vi "Calc_Waveform.vi"(1 "X-length":dbl, 5 "CamTolerance":dbl=1.1, 9 "frequency in":dbl=5000.0, 11 "error in":errorcluster, 12 "X-Delta":dbl) -> (4 "TriggerLineCamWavepoints":dbl[](array[numeric]), 6 "divisor out":i32, 8 "Array":u8[](array[numeric]), 15 "error out":errorcluster)   [LabVIEW 2011]
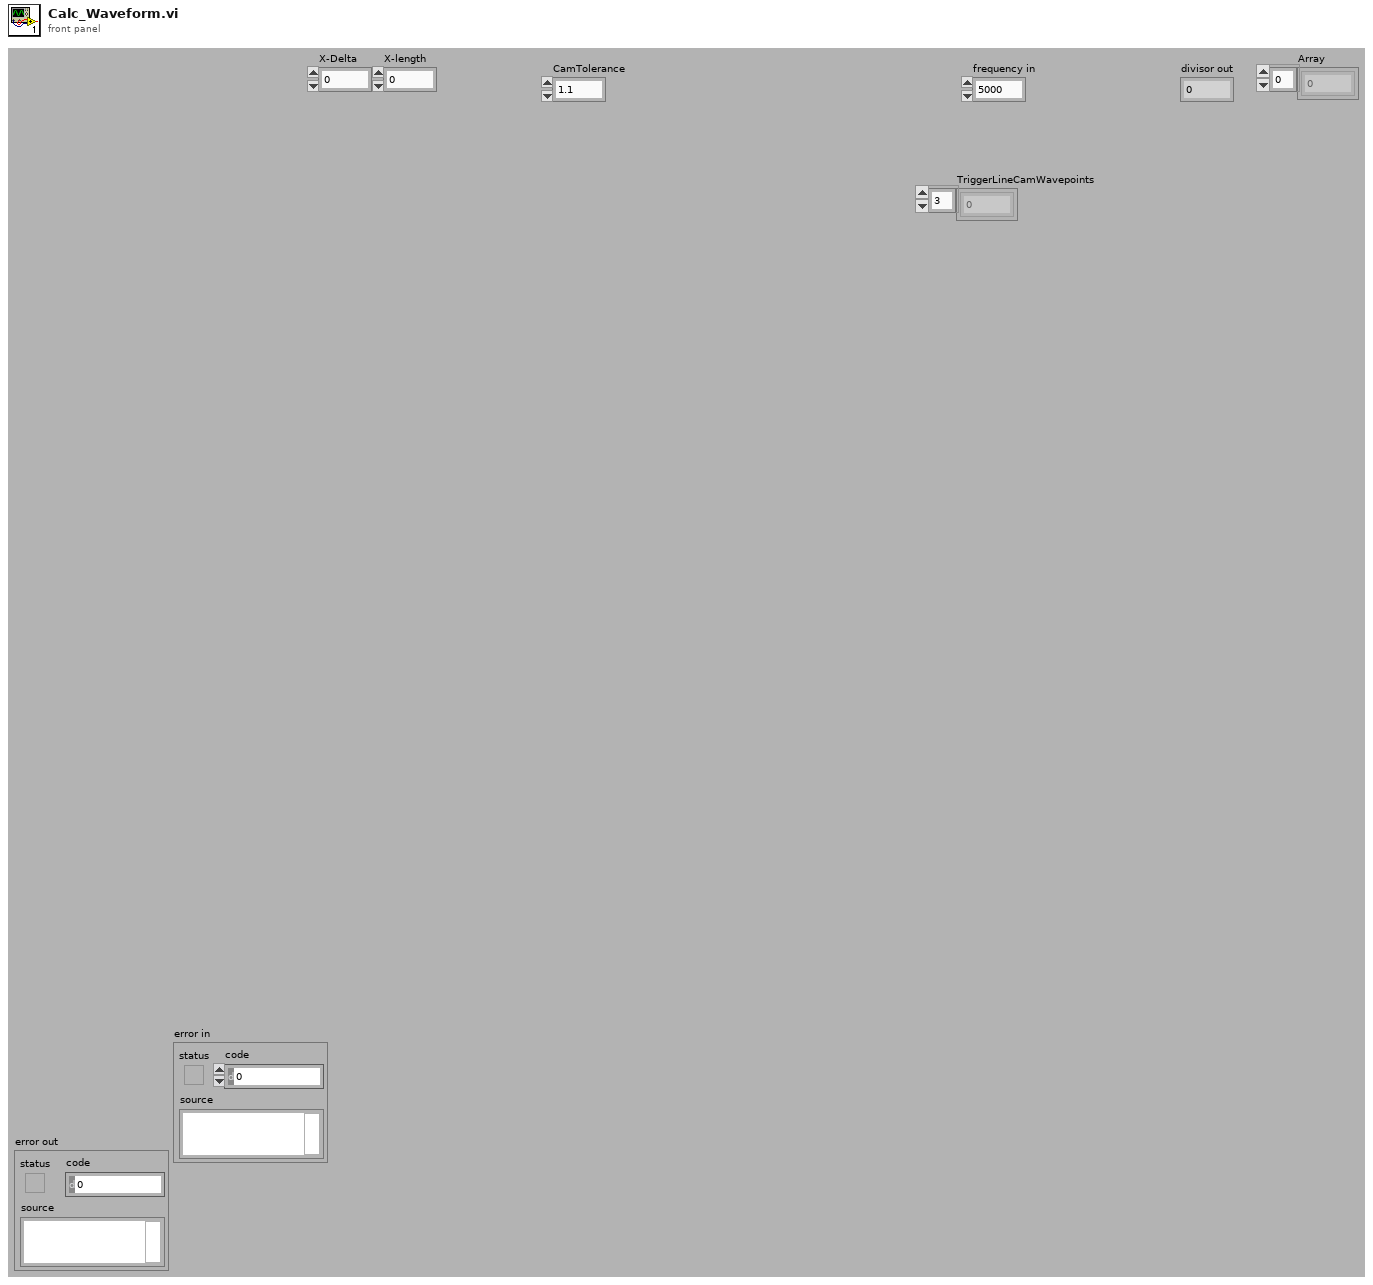
[diagram p1: front panel]
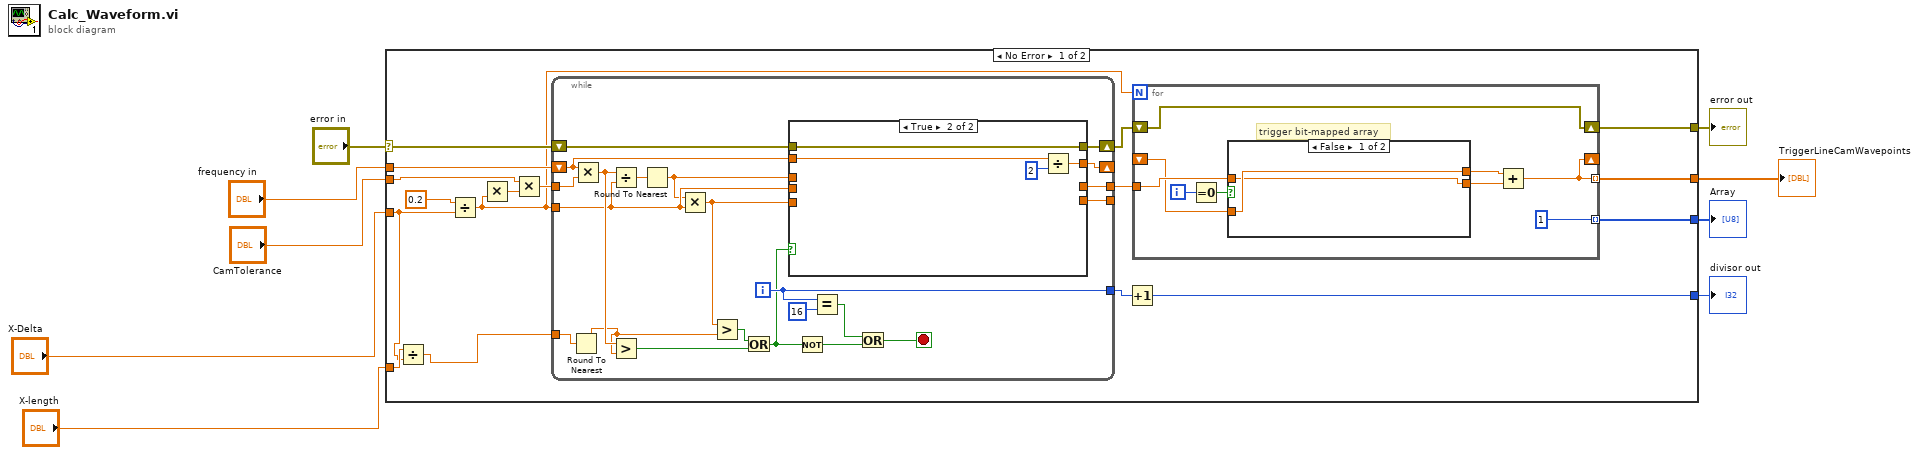
[diagram p0: block diagram]
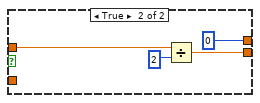
[diagram p2: hidden frame]
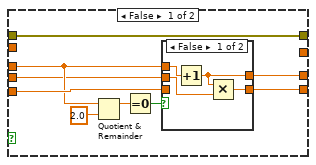
[diagram p3: hidden frame]
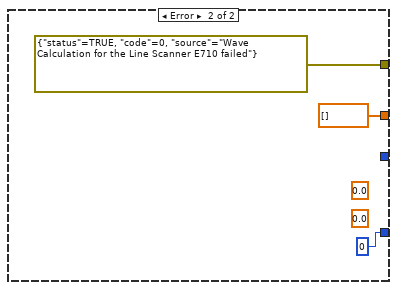
[diagram p5: hidden frame]
diagram:
  n1 = case shown="No Error" "error in" {
    selector: "error in" -> [w19 _]
    tunnel: "frequency in" -> [w26 _]
    tunnel: "CamTolerance" -> [w24 _]
    tunnel: [w21 errorcluster {"status"=TRUE, "code"=0, "source"="Wave Calculation for the Line Scanner E710 failed"} ("error IO")] -> w4
    tunnel: [w17 0] -> w7
    tunnel: [w18 dbl[] []] -> w5
    tunnel: [w15 _] -> w3
    tunnel: "X-Delta" -> [w11 _]
    tunnel: "X-length" -> [w12 _]
    frame No Error {
      n2 = Divide(x=w12, y=w11) -> (x/y=w10:dbl)
      n3 = Divide(x=0.2, y=w11) -> (x/y=w13:dbl)
      n4 = Multiply(y=w13) -> (x*y=w23:dbl)  [unwired: 1 in]
      n5 = Multiply(x=w24, y=w23) -> (x*y=w25:dbl)
      n6 = while {
        shift-right: [w61] -> _
        shift-left: w26 -> [w62]
        tunnel: w10 -> [w43]
        tunnel: w25 -> [w60]
        shift-right: [w58] -> w22
        shift-left: w19 -> [w59]
        tunnel: [w63] -> _
        tunnel: [w53] -> w16
        tunnel: w13 -> [w46]
        tunnel: [w44] -> w20
        i -> [w53]
        stop <- w56 stop-if-true
        n7 = Round To Nearest(number=w43) -> (nearest integer value=w42:dbl)
        n8 = Multiply(x=w62, y=w60) -> (x*y=w51:dbl)
        n9 = Divide(x=w51, y=w46) -> (x/y=w52:dbl)
        n10 = Greater?(x=w51, y=w42) -> (0:w49:bool)
        n11 = Round To Nearest(number=w52) -> (nearest integer value=w45:dbl)
        n12 = Multiply(x=w45, y=w46) -> (x*y=w47:dbl)
        n13 = Greater?(x=w47, y=w42) -> (0:w50:bool)
        n14 = Or(x=w50, y=w49) -> (x .or. y?=w48:bool)
        n15 = case shown="True" w48 {
          tunnel: w47 -> [w68 _]
          tunnel: [w67 _] -> w63
          tunnel: w62 -> [_ w82]
          tunnel: [_ w80] -> w61
          tunnel: w59 -> [w72 w79]
          tunnel: [w72 w79] -> w58
          tunnel: w45 -> [w66 _]
          tunnel: w46 -> [w65 _]
          tunnel: [w64 _] -> w44
          frame False {
            n16 = Quotient & Remainder(x=w66, y=2.0) -> (x-y*floor(x/y)=w70:dbl)  [unwired: 1 out]
            n17 = Equal To 0?(x=w70) -> (x = 0?=w69:bool)
            n18 = case shown="False" w69 {
              tunnel: w68 -> [_ w78]
              tunnel: [w75 w78] -> w67
              tunnel: w66 -> [w76 w77]
              tunnel: w65 -> [w74 _]
              tunnel: [w73 w77] -> w64
              frame False {
                n19 = Increment(x=w76) -> (x+1=w73:dbl)
                n20 = Multiply(x=w73, y=w74) -> (x*y=w75:dbl)
              }
              frame True {
              }
            }
          }
          frame True {
            n21 = Divide(x=w82, y=2) -> (x/y=w80:dbl)
          }
        }
        n22 = Not(x=w48) -> (.not. x?=w54:bool)
        n23 = Equal?(x=w53, y=16) -> (x = y?=w55:bool)
        n24 = Or(x=w55, y=w54) -> (x .or. y?=w56:bool)
      }
      n25 = Increment(x=w16) -> (x+1=w17:i32)
      n26 = for {
        N: w13 -> [_]
        shift-right: [w35] -> w21
        shift-left: w22 -> [w35]
        tunnel: w20 -> [w33]
        shift-right: [w29] -> _
        shift-left: _ -> [w32]
        tunnel: [w29] -> w18 mode=indexing
        tunnel: [1] -> w15 mode=indexing
        i -> [w28]
        # "trigger bit-mapped array"
        n27 = Equal To 0?(x=w28) -> (x = 0?=w34:bool)
        n28 = case shown="False" w34 {
          tunnel: w33 -> [w36 w40]
          tunnel: [w37 0] -> w31
          tunnel: w32 -> [w37 _]
          tunnel: [w36 w38] -> w30
          frame False {
          }
          frame True {
            n29 = Divide(x=w40, y=i8 2) -> (x/y=w38:dbl)
          }
        }
        n30 = Add(x=w31, y=w30) -> (x+y=w29:dbl)
      }
    }
    frame Error {
      (unwired) 0.0
      (unwired) 0.0
    }
  }
  "divisor out" <- w7
  "error out" <- w4
  "TriggerLineCamWavepoints" <- w5
  "Array" <- w3
